vi "capex 16 ch thermocouples.vi"(10 "Enum":enum16{"Mod1", "Mod2", "Mod3", "Mod4", "Mod5"}(ring)=enum."Mod5") -> ()   [LabVIEW 2013]
panel:
  in  "Autoscale y?":bool
  in  "Number of data points to display":dbl=10000.0
  in  "clear data":bool
  in  "Save new names":bool
  in  "Quit":bool
  out "Numeric 16":dbl
  out "Numeric 15":dbl
  out "Numeric 14":dbl
  out "Numeric 13":dbl
  out "Numeric 12":dbl
  out "Numeric 11":dbl
  out "Numeric 10":dbl
  out "Numeric 9":dbl
  out "Numeric 8":dbl=23.805375600154097
  out "Numeric 7":dbl=-55845.02175971931
  out "Numeric 6":dbl=-55845.02175971931
  out "Numeric 5":dbl=-55845.02175971931
  out "Numeric 4":dbl=-55859.71656674185
  out "Numeric 3":dbl=-55859.71656674185
  out "Numeric 2":dbl=-55859.71656674185
  out "Numeric":dbl=-55859.71656674185
  in  "String 18":string
  in  "String 17":string
  in  "String 16":string
  in  "String 15":string
  in  "String 14":string
  in  "String 13":string
  in  "String 12":string
  in  "String 11":string
  in  "String 10":string="Mod5TC8"
  in  "String 8":string="Mod5TC7"
  in  "String 7":string="Mod5TC6"
  in  "String 6":string="Mod5TC5"
  in  "String 5":string="Mod5TC4"
  in  "String 4":string="Mod5TC3"
  in  "String 3":string="Mod5TC2"
  in  "String 2":string="Mod5TC1"
  out "Temperature Chart 4":cluster{timestamp[], dbl[]}[](graph)
  # "X length"
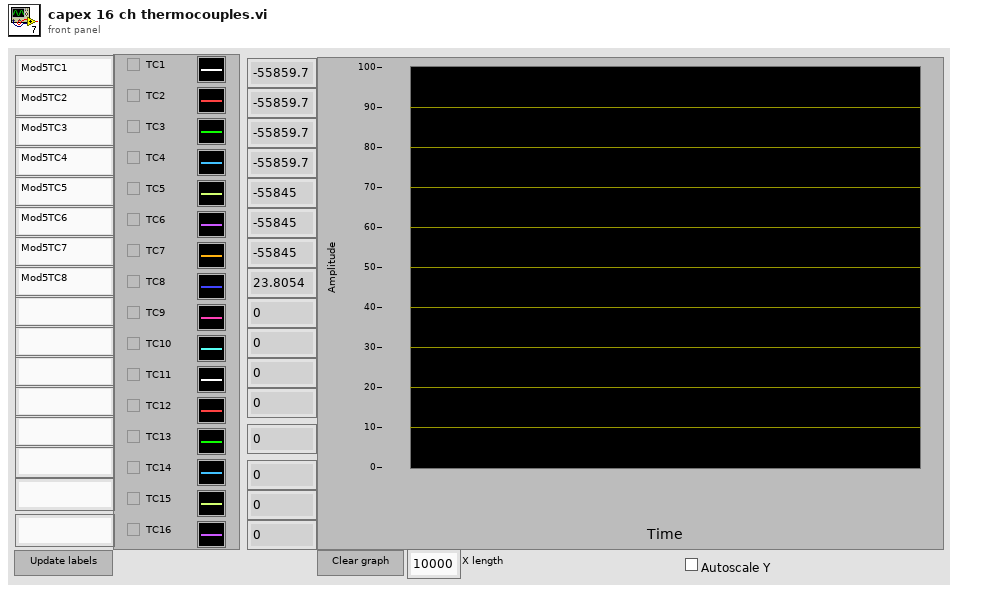
[diagram p1: front panel]
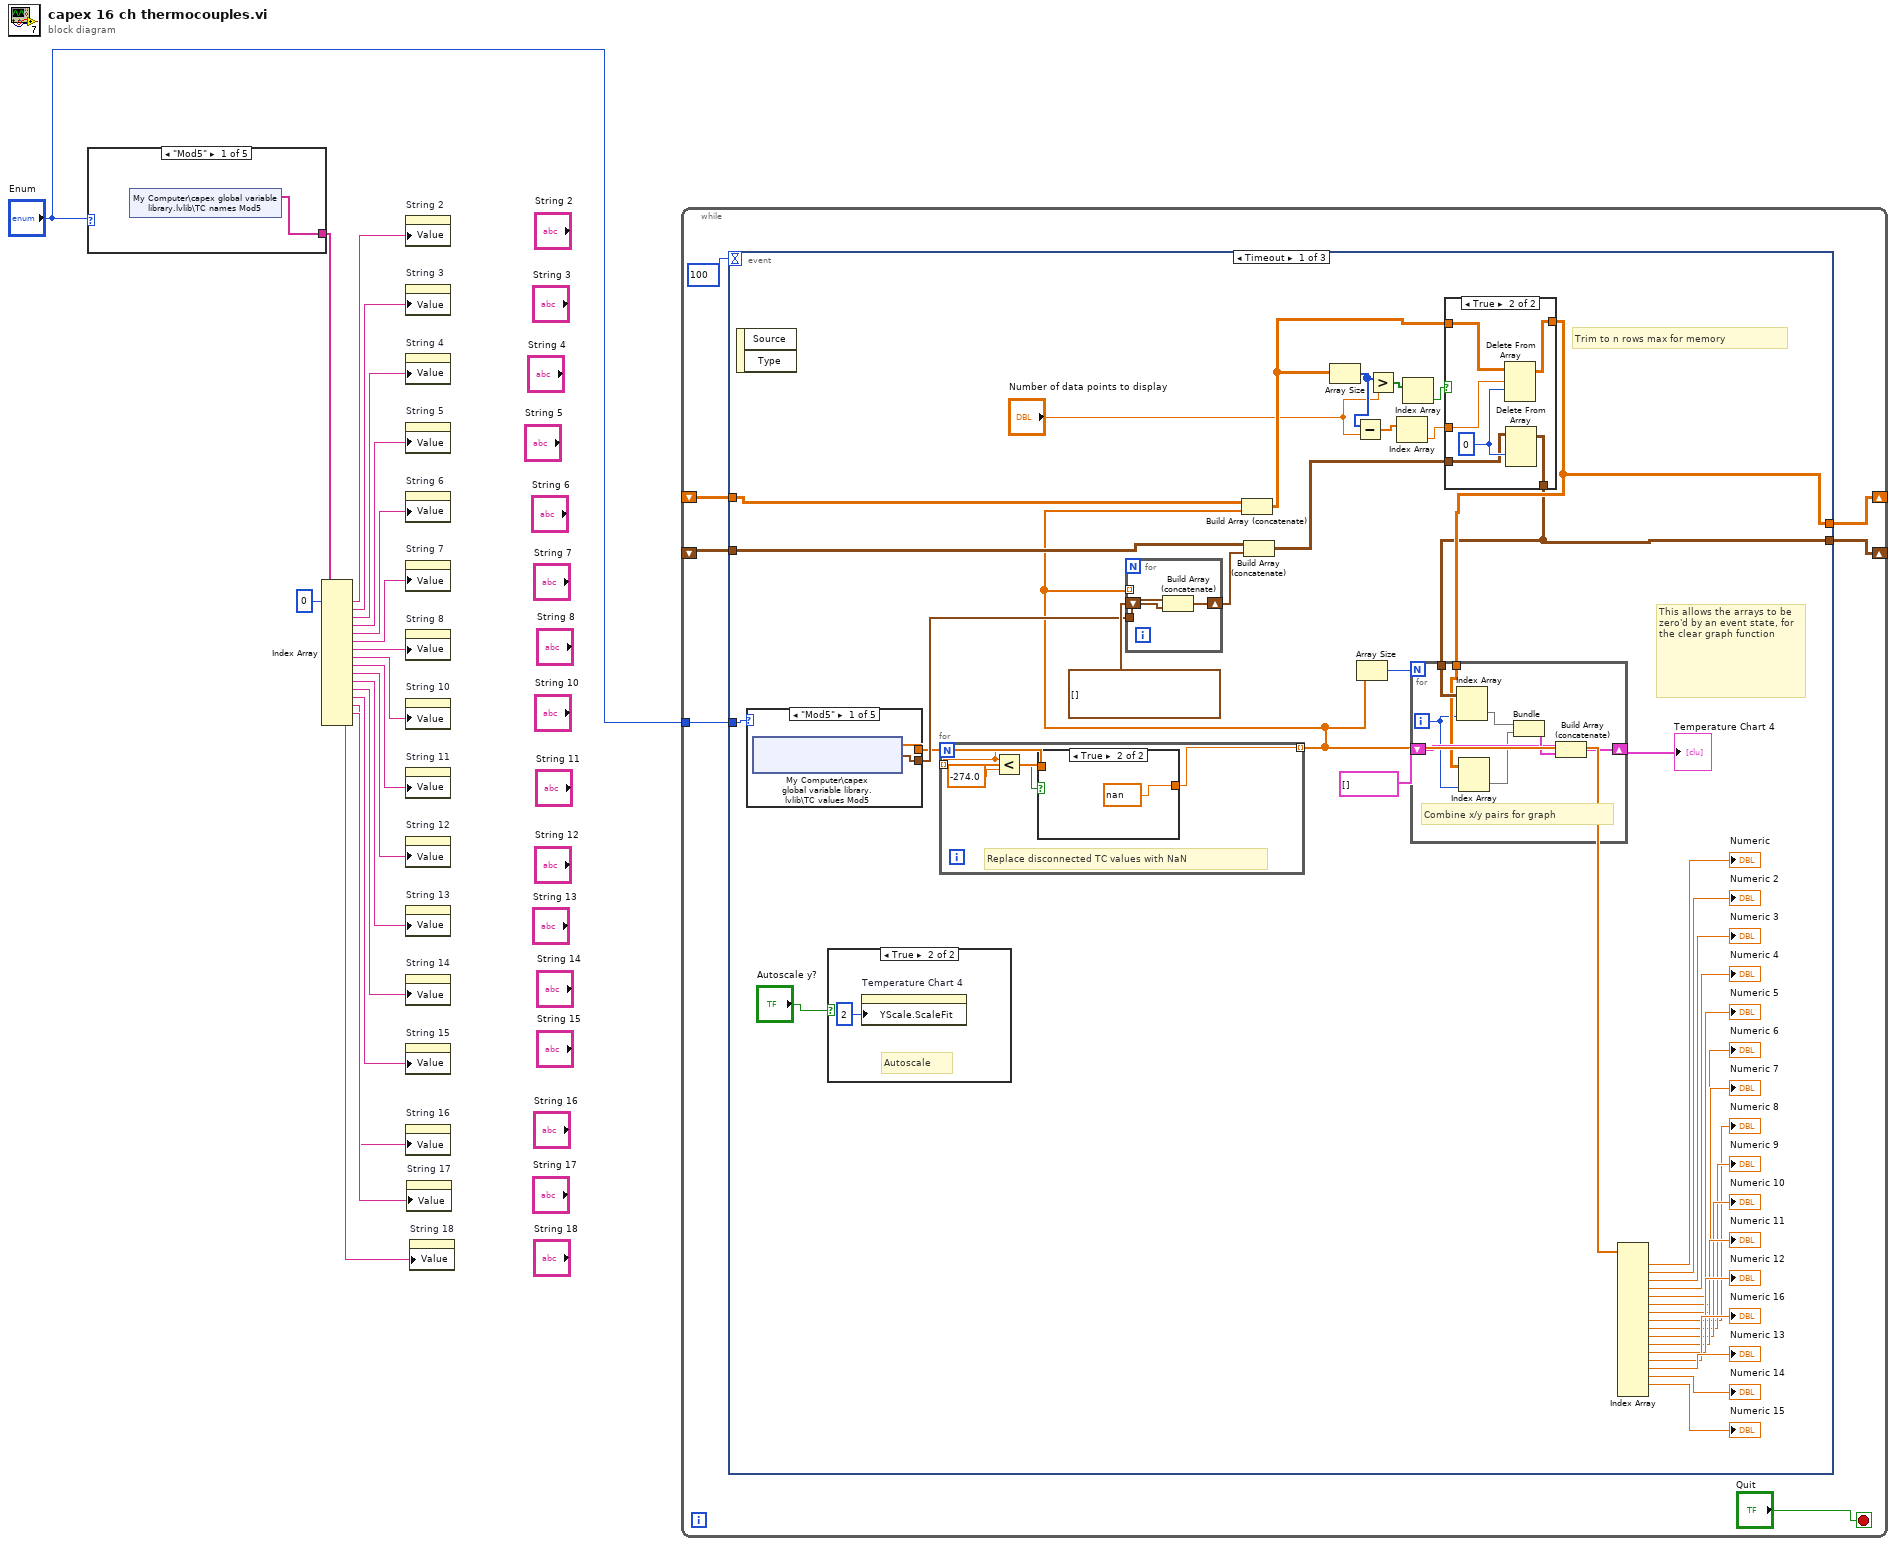
[diagram p0: block diagram]
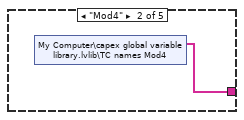
[diagram p2: hidden frame]
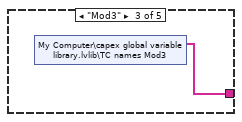
[diagram p3: hidden frame]
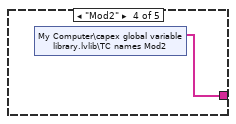
[diagram p4: hidden frame]
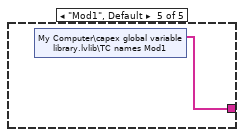
[diagram p5: hidden frame]
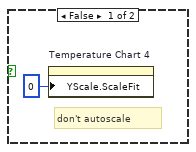
[diagram p6: hidden frame]
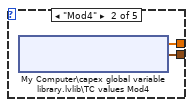
[diagram p9: hidden frame]
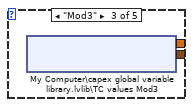
[diagram p10: hidden frame]
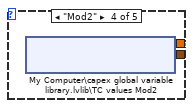
[diagram p11: hidden frame]
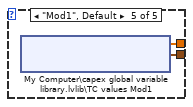
[diagram p12: hidden frame]
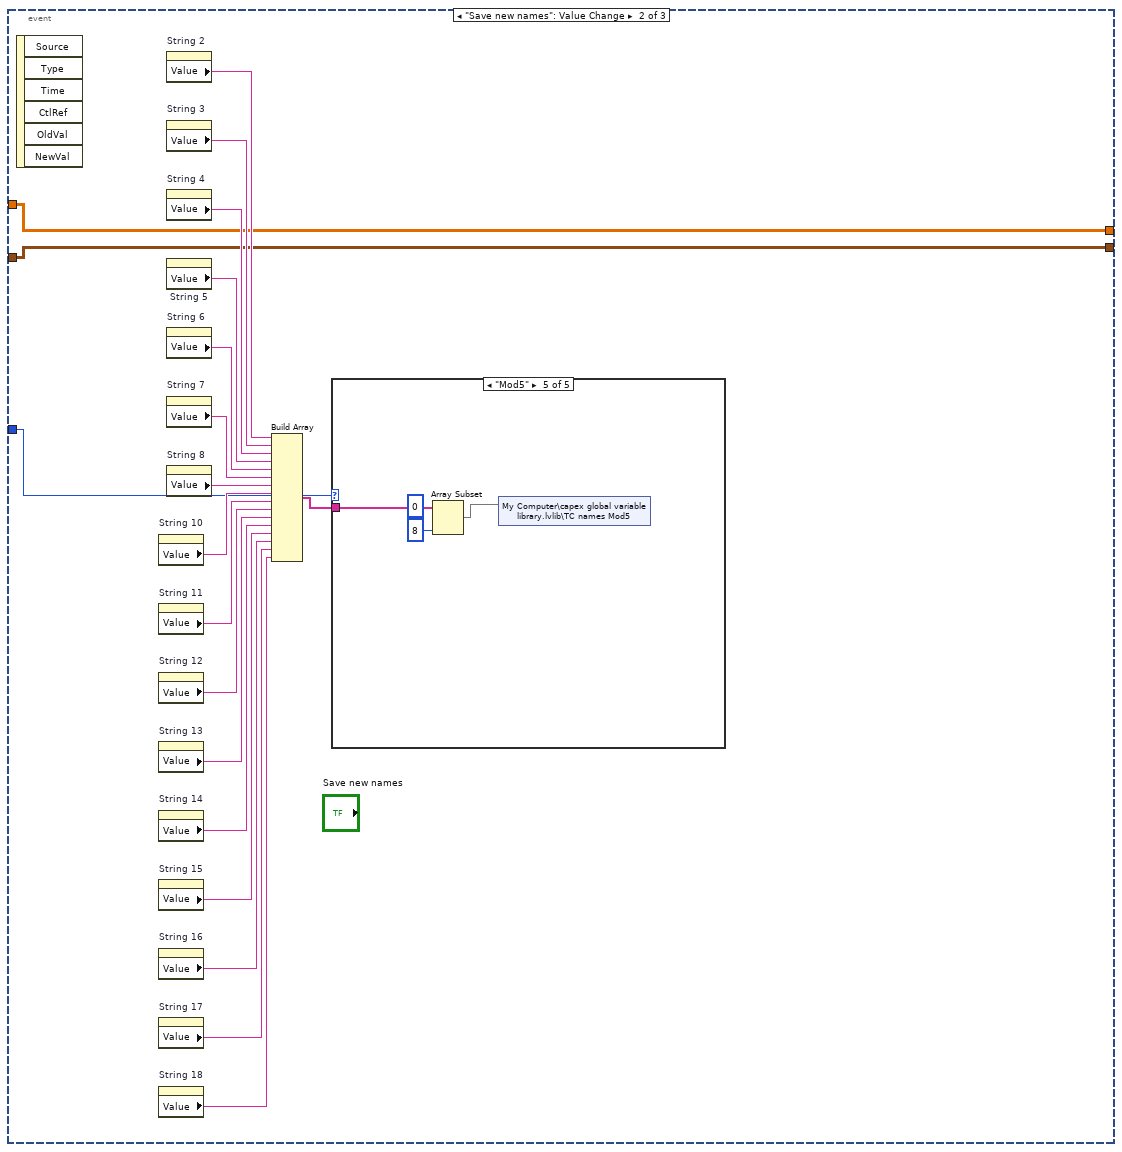
[diagram p13: hidden frame]
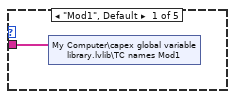
[diagram p14: hidden frame]
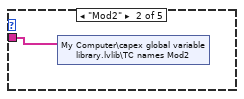
[diagram p15: hidden frame]
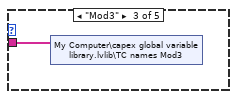
[diagram p16: hidden frame]
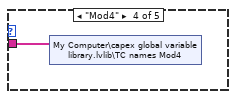
[diagram p17: hidden frame]
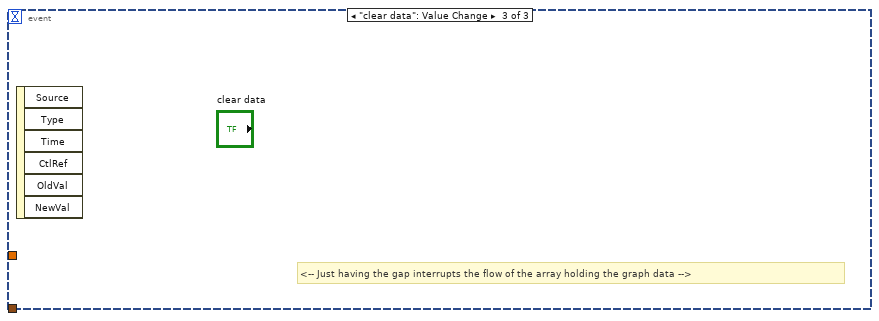
[diagram p18: hidden frame]
diagram:
  n1 = case shown="\"Mod5\"" "Enum" {
    tunnel: [w20 w21 w22 w23 w24] -> w2
    frame "Mod5" {
      n2 = shared-variable "My Computer\\capex global variable library.lvlib\\TC names Mod5"() -> (w20:string[])  [unwired: 1 in, 1 out]
    }
    frame "Mod4" {
      n3 = shared-variable "My Computer\\capex global variable library.lvlib\\TC names Mod4"() -> (w21:string[])  [unwired: 1 in, 1 out]
    }
    frame "Mod3" {
      n4 = shared-variable "My Computer\\capex global variable library.lvlib\\TC names Mod3"() -> (w22:string[])  [unwired: 1 in, 1 out]
    }
    frame "Mod2" {
      n5 = shared-variable "My Computer\\capex global variable library.lvlib\\TC names Mod2"() -> (w23:string[])  [unwired: 1 in, 1 out]
    }
    frame "Mod1", Default {
      n6 = shared-variable "My Computer\\capex global variable library.lvlib\\TC names Mod1"() -> (w24:string[])  [unwired: 1 in, 1 out]
    }
  }
  n7 = Index Array(array=w2, index #1=0 ("index")) -> (element #1=w3:string, element #2=w4:string, element #3=w5:string, element #4=w6:string, element #5=w7:string, element #6=w8:string, element #7=w9:string, element #8=w10:string, element #9=w11:string, element #10=w12:string, element #11=w13:string, element #12=w14:string, element #13=w15:string, element #14=w16:string, element #15=w18:string, element #16=w19:string)  [unwired: 15 in]
  n8 = property on="String 2" class="Str"("Value"=w3) -> ()  [unwired: 2 in, 2 out]
  n9 = property on="String 3" class="Str"("Value"=w4) -> ()  [unwired: 2 in, 2 out]
  n10 = property on="String 4" class="Str"("Value"=w5) -> ()  [unwired: 2 in, 2 out]
  n11 = property on="String 5" class="Str"("Value"=w6) -> ()  [unwired: 2 in, 2 out]
  n12 = property on="String 6" class="Str"("Value"=w7) -> ()  [unwired: 2 in, 2 out]
  n13 = property on="String 7" class="Str"("Value"=w8) -> ()  [unwired: 2 in, 2 out]
  n14 = property on="String 8" class="Str"("Value"=w9) -> ()  [unwired: 2 in, 2 out]
  n15 = property on="String 10" class="Str"("Value"=w10) -> ()  [unwired: 2 in, 2 out]
  n16 = property on="String 11" class="Str"("Value"=w11) -> ()  [unwired: 2 in, 2 out]
  n17 = property on="String 12" class="Str"("Value"=w12) -> ()  [unwired: 2 in, 2 out]
  n18 = property on="String 13" class="Str"("Value"=w13) -> ()  [unwired: 2 in, 2 out]
  n19 = property on="String 14" class="Str"("Value"=w14) -> ()  [unwired: 2 in, 2 out]
  n20 = property on="String 15" class="Str"("Value"=w15) -> ()  [unwired: 2 in, 2 out]
  n21 = property on="String 16" class="Str"("Value"=w16) -> ()  [unwired: 2 in, 2 out]
  n22 = property on="String 17" class="Str"("Value"=w18) -> ()  [unwired: 2 in, 2 out]
  n23 = property on="String 18" class="Str"("Value"=w19) -> ()  [unwired: 2 in, 2 out]
  n24 = while {
    shift-right: [w25] -> _
    shift-left: _ -> [w27]
    shift-right: [w26] -> _
    shift-left: _ -> [w28]
    tunnel: "Enum" -> [w29]
    stop <- "Quit" stop-if-true
    n25 = event shown="[0] Timeout" {
      selector: _ -> [_ _ _]
      dyn-events: _ -> [_ _ _]
      timeout: 100 -> [_ _ _]
      tunnel: w29 -> [w40 w109 _]
      tunnel: w28 -> [w39 w108 _]
      tunnel: w27 -> [w38 w107 _]
      tunnel: [w37 w108 _] -> w26
      tunnel: [w36 w107 _] -> w25
      event Timeout {
        # "This allows the arrays to be zero'd by an event state, for the clear graph function"
        # "Trim to n rows max for memory"
        n26 = event-data() -> ()  [unwired: 1 in, 2 out]
        n27 = case shown="\"Mod5\"" w40 {
          tunnel: [w98 w100 w102 w104 w106] -> w35
          tunnel: [w97 w99 w101 w103 w105] -> w41
          frame "Mod5" {
            n28 = shared-variable "My Computer\\capex global variable library.lvlib\\TC values Mod5"() -> (w98:dbl[], w97:timestamp)  [unwired: 1 in, 1 out]
          }
          frame "Mod4" {
            n29 = shared-variable "My Computer\\capex global variable library.lvlib\\TC values Mod4"() -> (w100:dbl[], w99:timestamp)  [unwired: 1 in, 1 out]
          }
          frame "Mod3" {
            n30 = shared-variable "My Computer\\capex global variable library.lvlib\\TC values Mod3"() -> (w102:dbl[], w101:timestamp)  [unwired: 1 in, 1 out]
          }
          frame "Mod2" {
            n31 = shared-variable "My Computer\\capex global variable library.lvlib\\TC values Mod2"() -> (w104:dbl[], w103:timestamp)  [unwired: 1 in, 1 out]
          }
          frame "Mod1", Default {
            n32 = shared-variable "My Computer\\capex global variable library.lvlib\\TC values Mod1"() -> (w106:dbl[], w105:timestamp)  [unwired: 1 in, 1 out]
          }
        }
        n33 = case shown="True" "Autoscale y?" {
          frame False {
            # "don't autoscale"
            n34 = property on="Temperature Chart 4" class="XYGraph (strict)"("YScale.ScaleFit"=u8 0 ("Y Scale.Scale Fit")) -> ()  [unwired: 2 in, 2 out]
          }
          frame True {
            # "Autoscale"
            n35 = property on="Temperature Chart 4" class="XYGraph (strict)"("YScale.ScaleFit"=u8 2 ("Y Scale.Scale Fit")) -> ()  [unwired: 2 in, 2 out]
          }
        }
        n36 = for {
          tunnel: [w73] -> w32 mode=indexing
          tunnel: w35 -> [w72] mode=indexing
          # "Replace disconnected TC values with NaN"
          n37 = Less?(x=w72, y=-274.0) -> (x < y?=w74:bool)
          n38 = case shown="True" w74 {
            tunnel: [w76 nan] -> w73
            tunnel: w72 -> [w76 _]
            frame False {
            }
            frame True {
            }
          }
        }
        n39 = for {
          tunnel: w32 -> [_] mode=indexing
          shift-right: [w96] -> w43
          shift-left: timestamp[] [] -> [w94]
          tunnel: w41 -> [w95]
          n40 = Build Array (concatenate)(w95, w94) -> (w96:timestamp[])
        }
        n41 = Build Array (concatenate)(w39, w32) -> (w52:dbl[][])
        n42 = Build Array (concatenate)(w38, w43) -> (w53:timestamp[][])
        n43 = Array Size(array=w52) -> (size(s)=w47:i32[])
        n44 = Subtract(x=w47, y="Number of data points to display") -> (x-y=w50:dbl[])
        n45 = Array Size(array=w32) -> (size(s)=w44:i32)
        n46 = Greater?(x=w47, y="Number of data points to display") -> (0:w48:bool[])
        n47 = Index Array(array=w50) -> (element=w51:dbl)  [unwired: 1 in]
        n48 = Index Array(array=w48) -> (element=w49:bool)  [unwired: 1 in]
        n49 = case shown="True" w49 {
          tunnel: [w79 w83] -> w37
          tunnel: w52 -> [w79 w85]
          tunnel: w51 -> [_ w84]
          tunnel: w53 -> [w78 w81]
          tunnel: [w78 w80] -> w36
          frame False {
          }
          frame True {
            w82 = 0 ("index")
            n50 = Delete From Array(array=w85, length=w84, index (row)=w82) -> (array with subset deleted=w83:dbl[][])  [unwired: 1 in, 1 out]
            n51 = Delete From Array(array=w81, index (row)=w82) -> (array with subset deleted=w80:timestamp[][])  [unwired: 2 in, 1 out]
          }
        }
        n52 = for {
          N: w44 -> [_]
          tunnel: w37 -> [w87]
          tunnel: w36 -> [w90]
          shift-right: [w92] -> w45
          shift-left: cluster{timestamp[], dbl[]}[] [] -> [w91]
          i -> [w86]
          # "Combine x/y pairs for graph"
          n53 = Index Array(array=w90, index (col)=w86) -> (element=w89:timestamp[])  [unwired: 1 in]
          n54 = Index Array(array=w87, index (col)=w86) -> (element=w88:dbl[])  [unwired: 1 in]
          n55 = Bundle(w89, w88) -> (w93:cluster{timestamp[], dbl[]})  [unwired: 1 in]
          n56 = Build Array (concatenate)(w91, w93) -> (w92:cluster{timestamp[], dbl[]}[])
        }
        "Temperature Chart 4" <- w45
        n57 = Index Array(array=w32) -> (element #1=→"Numeric":dbl, element #2=→"Numeric 2":dbl, element #3=→"Numeric 3":dbl, element #4=→"Numeric 4":dbl, element #5=→"Numeric 5":dbl, element #6=→"Numeric 6":dbl, element #7=→"Numeric 7":dbl, element #8=→"Numeric 8":dbl, element #9=→"Numeric 9":dbl, element #10=→"Numeric 10":dbl, element #11=→"Numeric 11":dbl, element #12=→"Numeric 12":dbl, element #13=→"Numeric 16":dbl, element #14=→"Numeric 13":dbl, element #15=→"Numeric 14":dbl, element #16=→"Numeric 15":dbl)  [unwired: 17 in, 1 out]
      }
      event "Save new names": Value Change {
        n58 = event-data() -> ()  [unwired: 1 in, 6 out]
        n59 = property on="String 10" class="Str"() -> ("Value"=w119:string)  [unwired: 2 in, 2 out]
        n60 = property on="String 11" class="Str"() -> ("Value"=w118:string)  [unwired: 2 in, 2 out]
        n61 = property on="String 12" class="Str"() -> ("Value"=w117:string)  [unwired: 2 in, 2 out]
        n62 = property on="String 13" class="Str"() -> ("Value"=w116:string)  [unwired: 2 in, 2 out]
        n63 = property on="String 14" class="Str"() -> ("Value"=w115:string)  [unwired: 2 in, 2 out]
        n64 = property on="String 15" class="Str"() -> ("Value"=w114:string)  [unwired: 2 in, 2 out]
        n65 = property on="String 16" class="Str"() -> ("Value"=w113:string)  [unwired: 2 in, 2 out]
        n66 = property on="String 17" class="Str"() -> ("Value"=w112:string)  [unwired: 2 in, 2 out]
        n67 = property on="String 18" class="Str"() -> ("Value"=w111:string)  [unwired: 2 in, 2 out]
        n68 = property on="String 2" class="Str"() -> ("Value"=w126:string)  [unwired: 2 in, 2 out]
        n69 = property on="String 3" class="Str"() -> ("Value"=w125:string)  [unwired: 2 in, 2 out]
        n70 = property on="String 4" class="Str"() -> ("Value"=w124:string)  [unwired: 2 in, 2 out]
        n71 = property on="String 5" class="Str"() -> ("Value"=w123:string)  [unwired: 2 in, 2 out]
        n72 = property on="String 6" class="Str"() -> ("Value"=w122:string)  [unwired: 2 in, 2 out]
        n73 = property on="String 7" class="Str"() -> ("Value"=w121:string)  [unwired: 2 in, 2 out]
        n74 = property on="String 8" class="Str"() -> ("Value"=w120:string)  [unwired: 2 in, 2 out]
        n75 = Build Array(w126, w125, w124, w123, w122, w121, w120, w119, w118, w117, w116, w115, w114, w113, w112, w111) -> (w110:string[])
        n76 = case shown="\"Mod5\"" w109 {
          tunnel: w110 -> [w127 w128 w129 w130 w134]
          frame "Mod1", Default {
            n77 = shared-variable "My Computer\\capex global variable library.lvlib\\TC names Mod1"(w127) -> ()  [unwired: 1 in, 1 out]
          }
          frame "Mod2" {
            n78 = shared-variable "My Computer\\capex global variable library.lvlib\\TC names Mod2"(w128) -> ()  [unwired: 1 in, 1 out]
          }
          frame "Mod3" {
            n79 = shared-variable "My Computer\\capex global variable library.lvlib\\TC names Mod3"(w129) -> ()  [unwired: 1 in, 1 out]
          }
          frame "Mod4" {
            n80 = shared-variable "My Computer\\capex global variable library.lvlib\\TC names Mod4"(w130) -> ()  [unwired: 1 in, 1 out]
          }
          frame "Mod5" {
            n81 = Array Subset(array=w134, index=0, length=8) -> (w131:string[])
            n82 = shared-variable "My Computer\\capex global variable library.lvlib\\TC names Mod5"(w131) -> ()  [unwired: 1 in, 1 out]
          }
        }
      }
      event "clear data": Value Change {
        # "<-- Just having the gap interrupts the flow of the array holding the graph data -->"
        n83 = event-data() -> ()  [unwired: 1 in, 6 out]
      }
    }
  }
